vi "Square Wave.vi"(0 "samples":i32=128, 1 "reset phase":bool=TRUE, 2 "amplitude":dbl=1.0 format="%0.2f", 3 "frequency":dbl=0.0078125 format="%0.4e", 4 "duty cycle (%)":dbl=50.0 format="%0.2f", 5 "phase in":dbl format="%0.2f") -> (6 "square wave":dbl[](array[numeric]), 7 "phase out":dbl format="%0.2e", 8 "error":i32)   [LabVIEW 2017, in "NI_AALBase.lvlib"]
doc: "Generates an array containing a square wave."
uses:
  NI_AALBase.lvlib
  <resource>/lvanlys.dll
panel:
  # "Square Wave"
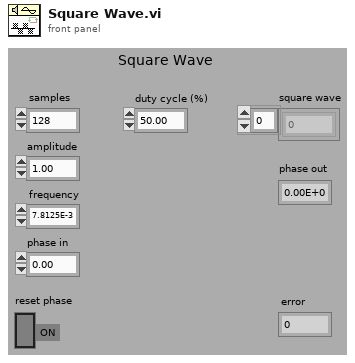
[diagram p1: front panel]
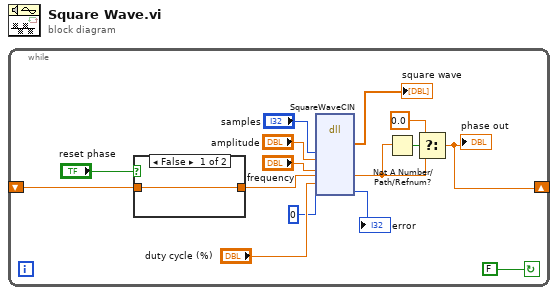
[diagram p0: block diagram]
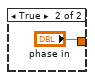
[diagram p2: hidden frame]
diagram:
  n1 = while {
    shift-left: _ -> [w14]
    shift-right: [w10] -> _
    stop <- FALSE continue-if-true
    n2 = case shown="False" "reset phase" {
      tunnel: [w16 "phase in"] -> w8
      tunnel: w14 -> [w16 _]
      frame False {
      }
      frame True {
      }
    }
    n3 = dll-call lib="C:/Program Files (x86)/National Instruments/LabVIEW 2017/resource/lvanlys.*" fn="SquareWaveCIN"("samples"="samples", "amplitude"="amplitude", "frequency"="frequency", "phase in"=w8, "duty cycle (%)"="duty cycle (%)", "output param"=0) -> ("square wave"=→"square wave":dbl[], "phase in"=w7:dbl, "output param"=→"error":i32)  [unwired: 9 in, 2 out]
    n4 = Not A Number/Path/Refnum?(number/path/refnum=w7) -> (NaN/Path/Refnum?=w12:bool)
    n5 = Select(t=0.0, s=w12, f=w7) -> (s? t:f=w10:dbl)
    "phase out" <- w10
  }
